vi "V50 Report Shot Table (SubVI).vi"(0 "NI_report in":refnum<class "NI_report.lvclass">, 5 "SampleID":string, 11 "error in (no error)":errorcluster) -> (4 "NI_report out":refnum<class "NI_report.lvclass">, 15 "error out":errorcluster)   [LabVIEW 2015]
uses:
  <vilib>/Utility/NIReport.llb/NI_report.lvclass
  <vilib>/Utility/NIReport.llb/Excel/NI_Excel.lvclass
panel:
  out "BFDs":string[][](array[string])
  out "V50s":string[][](array[string])
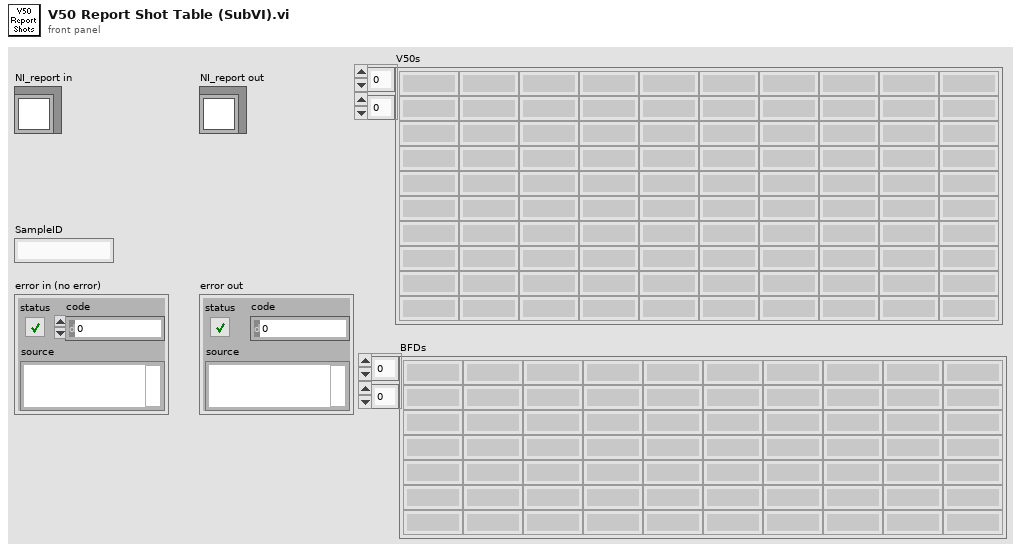
[diagram p1: front panel]
types:
  T1 = enum16{"Standard Report", "HTML", "Word", "Excel"}
  T2 = cluster{"position (excel)":cluster{"row":i32, "column":i32}, "name (excel)":string, "bookmark (word)":string}
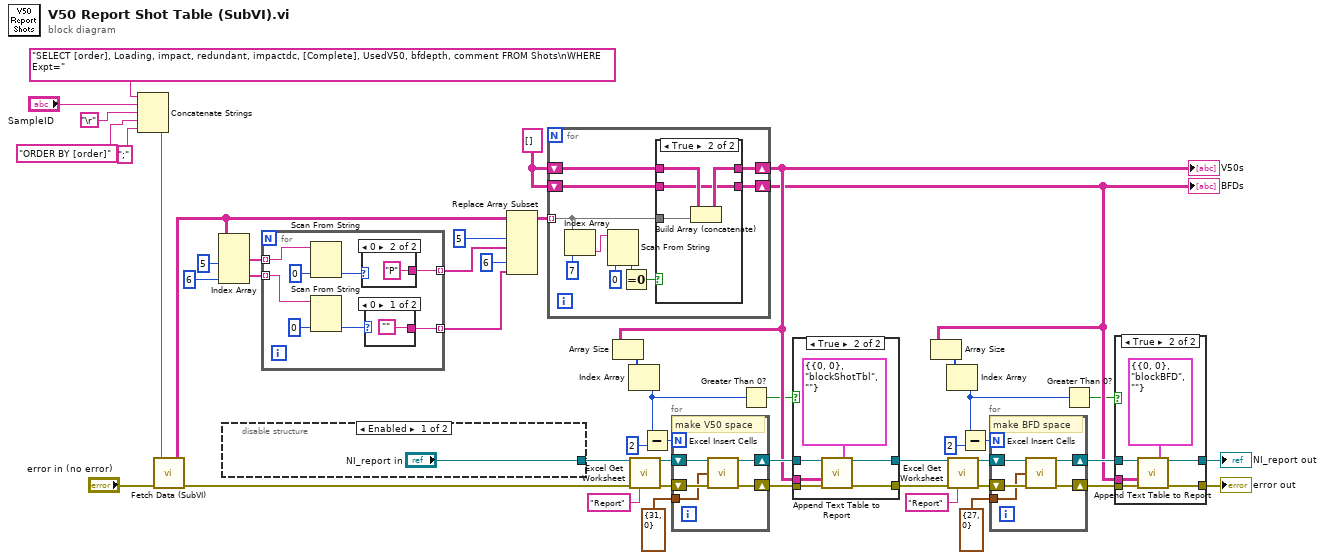
[diagram p0: block diagram]
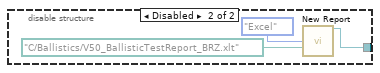
[diagram p4: hidden frame]
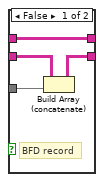
[diagram p5: hidden frame]
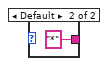
[diagram p6: hidden frame]
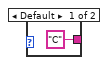
[diagram p7: hidden frame]
diagram:
  w22 = string[][] [] ("output array")
  n1 = Concatenate Strings("SELECT [order], Loading, impact, redundant, impactdc, [Complete], UsedV50, bfdepth, comment FROM Shots\nWHERE Expt=" ("query string"), "SampleID", "\r", "ORDER BY [order]" ("query string"), ";" ("string")) -> (w47:string)
  n2 = call "Fetch Data (SubVI).vi"("error IN"="error in (no error)", "query string"=w47) -> ("error OUT"=w29:errorcluster, "recordset data"=w42:string[][])  [unwired: 4 out]
  n3 = Index Array(array=w42, index (col) #1=5 ("index (row)"), index (col) #2=6 ("index (col)")) -> (element #1=w40:string[], element #2=w36:string[])  [unwired: 2 in]
  n4 = disable-structure shown="Enabled" {
    disable-tunnel: ["NI_report in" w50] -> w31
    frame Enabled {
    }
    frame Disabled {
      n5 = call <vilib>:"New Report.vi"("report type"=T1."Excel", "template (empty)"=path "C:/Ballistics/V50_BallisticTestReport_BRZ.xlt" ("Custom Template")) -> ("report out"=w50:refnum<class "NI_report.lvclass">)  [unwired: 12 in, 1 out]
    }
  }
  n6 = for {
    tunnel: [w60] -> w41 mode=indexing
    tunnel: w40 -> [w59] mode=indexing
    tunnel: w36 -> [w55] mode=indexing
    tunnel: [w54] -> w34 mode=indexing
    n7 = Scan From String(input string=w59, default 1=0 ("default value 1")) -> (output 1=w57:i32)  [unwired: 3 in, 3 out]
    n8 = Scan From String(input string=w55, default 1=0 ("default value 1")) -> (output 1=w56:i32)  [unwired: 3 in, 3 out]
    n9 = case shown="0" w57 {
      tunnel: ["C" "P"] -> w60
      frame Default {
      }
      frame 0 {
      }
    }
    n10 = case shown="0" w56 {
      tunnel: ["" ("Empty String Constant") "*"] -> w54
      frame 0 {
      }
      frame Default {
      }
    }
  }
  n11 = Replace Array Subset(array=w42, new element #1=w41, index (col) #1=5 ("index (row)"), new element #2=w34, index (col) #2=6 ("index (col)")) -> (w23:string[][])  [unwired: 2 in]
  n12 = for {
    tunnel: w23 -> [w69] mode=indexing
    shift-right: [w68] -> w11
    shift-left: w22 -> [w66]
    shift-right: [w67] -> w8
    shift-left: w22 -> [w65]
    n13 = Index Array(array=w69, index=7 ("disabled index (col)")) -> (element=w73:string)
    n14 = Scan From String(input string=w73, default 1=0 ("default value 1")) -> (output 1=w71:i32)  [unwired: 3 in, 3 out]
    n15 = Equal To 0?(x=w71) -> (x = 0?=w70:bool)
    n16 = case shown="True" w70 {
      tunnel: w69 -> [w75 w79]
      tunnel: [w78 w82] -> w68
      tunnel: [w77 w80] -> w67
      tunnel: w66 -> [w78 w81]
      tunnel: w65 -> [w76 w80]
      frame False {
        # "BFD record"
        n17 = Build Array (concatenate)(w76, w75) -> (w77:string[][])
      }
      frame True {
        n18 = Build Array (concatenate)(w81, w79) -> (w82:string[][])
      }
    }
  }
  "V50s" <- w11
  "BFDs" <- w8
  n19 = Array Size(array=w11) -> (size(s)=w19:i32[])
  n20 = Index Array(array=w19) -> (element=w4:i32)  [unwired: 1 in]
  n21 = call <vilib>:"Excel Get Worksheet.vi"("report in"=w31, "error in (no error)"=w29, "name (\"\")"="Report" ("name (\"\")")) -> ("report out"=w30:refnum<class "NI_report.lvclass">, "error out"=w28:errorcluster)  [unwired: 11 in]
  n22 = Subtract(x=w4, y=2) -> (x-y=w24:i32)
  n23 = for {
    N: w24 -> [_]
    shift-right: [w84] -> w32
    shift-left: w30 -> [w87]
    shift-right: [w85] -> w33
    shift-left: w28 -> [w86]
    tunnel: cluster{"row":i32, "column":i32} {"row"=31, "column"=0} ("start (0, 0)") -> [w83]
    # "make V50 space"
    n24 = call <vilib>:"Excel Insert Cells.vi"("report in"=w87, "start (0, 0)"=w83, "error in (no error)"=w86) -> ("report out"=w84:refnum<class "NI_report.lvclass">, "error out"=w85:errorcluster)  [unwired: 11 in]
  }
  n25 = Greater Than 0?(x=w4) -> (x > 0?=w3:bool)
  n26 = case shown="True" w3 {
    tunnel: w33 -> [w88 w94]
    tunnel: w32 -> [w89 w93]
    tunnel: w11 -> [_ w92]
    tunnel: [w89 w91] -> w10
    tunnel: [w88 w90] -> w9
    frame False {
    }
    frame True {
      n27 = call-dynamic "Append Text Table to Report.vi"("report in"=w93, "MS Office parameters"=T2 {"position (excel)"={"row"=0, "column"=0}, "name (excel)"="blockShotTbl", "bookmark (word)"=""}, "text data"=w92, "error in (no error)"=w94) -> ("report out"=w91:refnum<class "NI_report.lvclass">, "error out"=w90:errorcluster)  [unwired: 8 in, 2 out]
    }
  }
  n28 = Array Size(array=w8) -> (size(s)=w18:i32[])
  n29 = Index Array(array=w18) -> (element=w2:i32)  [unwired: 1 in]
  n30 = call <vilib>:"Excel Get Worksheet.vi"("report in"=w10, "error in (no error)"=w9, "name (\"\")"="Report" ("name (\"\")")) -> ("report out"=w14:refnum<class "NI_report.lvclass">, "error out"=w15:errorcluster)  [unwired: 11 in]
  n31 = Subtract(x=w2, y=2) -> (x-y=w5:i32)
  n32 = for {
    N: w5 -> [_]
    shift-right: [w97] -> w13
    shift-left: w14 -> [w100]
    shift-right: [w98] -> w12
    shift-left: w15 -> [w99]
    tunnel: cluster{"row":i32, "column":i32} {"row"=27, "column"=0} ("start (0, 0)") -> [w96]
    # "make BFD space"
    n33 = call <vilib>:"Excel Insert Cells.vi"("report in"=w100, "start (0, 0)"=w96, "error in (no error)"=w99) -> ("report out"=w97:refnum<class "NI_report.lvclass">, "error out"=w98:errorcluster)  [unwired: 11 in]
  }
  n34 = Greater Than 0?(x=w2) -> (x > 0?=w1:bool)
  n35 = case shown="True" w1 {
    tunnel: [w102 w107] -> w21
    tunnel: [w101 w106] -> w20
    tunnel: w13 -> [w102 w105]
    tunnel: w12 -> [w101 w104]
    tunnel: w8 -> [_ w103]
    frame False {
    }
    frame True {
      n36 = call-dynamic "Append Text Table to Report.vi"("report in"=w105, "MS Office parameters"=T2 {"position (excel)"={"row"=0, "column"=0}, "name (excel)"="blockBFD", "bookmark (word)"=""}, "text data"=w103, "error in (no error)"=w104) -> ("report out"=w107:refnum<class "NI_report.lvclass">, "error out"=w106:errorcluster)  [unwired: 8 in, 2 out]
    }
  }
  "error out" <- w20
  "NI_report out" <- w21
